vi "FRC-Traj-Lib-timer-test.vi"() -> ()   [LabVIEW 2019]
uses:
  <vilib>/Rock Robotics/WPI/ThirdParty/JAS_Junk/TrajLib/Trajectory_Library.lvlib
panel:
  in  "Tab Control":enum32{"Control Panel", "Logic"}(tab)
  in  "Reset TImer":bool
  in  "Stop Timer":bool
  in  "Start Timer":bool
  out "Trend":cluster{"CurrentTImer":dbl, "CurrentTImer":dbl}(graph)
  out "Expired":bool
  out "Timer 2":dbl
  out "Timer 1":dbl
  # "Timer Test"
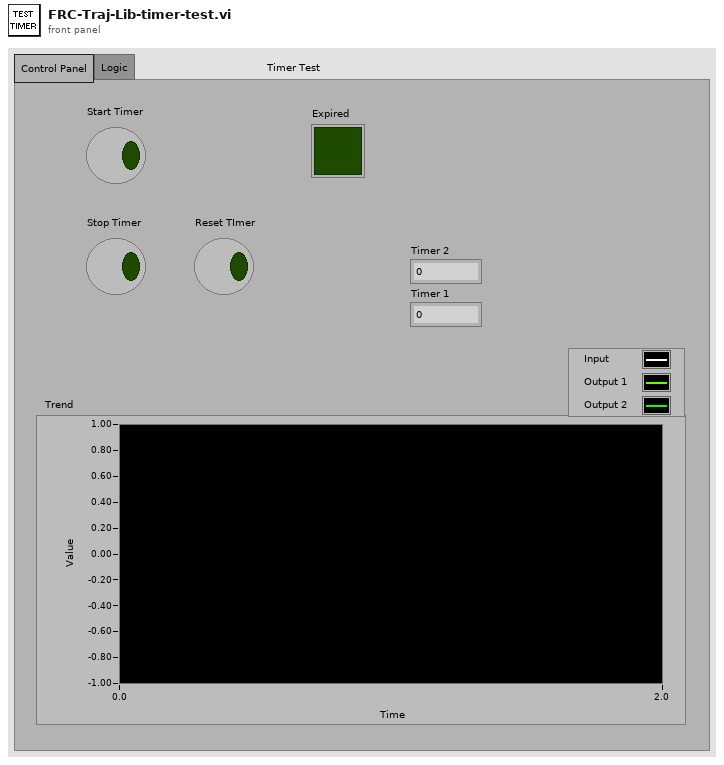
[diagram p1: front panel]
types:
  T1 = typedef "Trajectory_Library.lvlib/TIMER.ctl" = cluster{"StartTime":dbl, "Accumulated TIme":dbl, "Running":bool, "semaphore":T2}
  T2 = typedef "Semaphore RefNum" = refnum<k1>
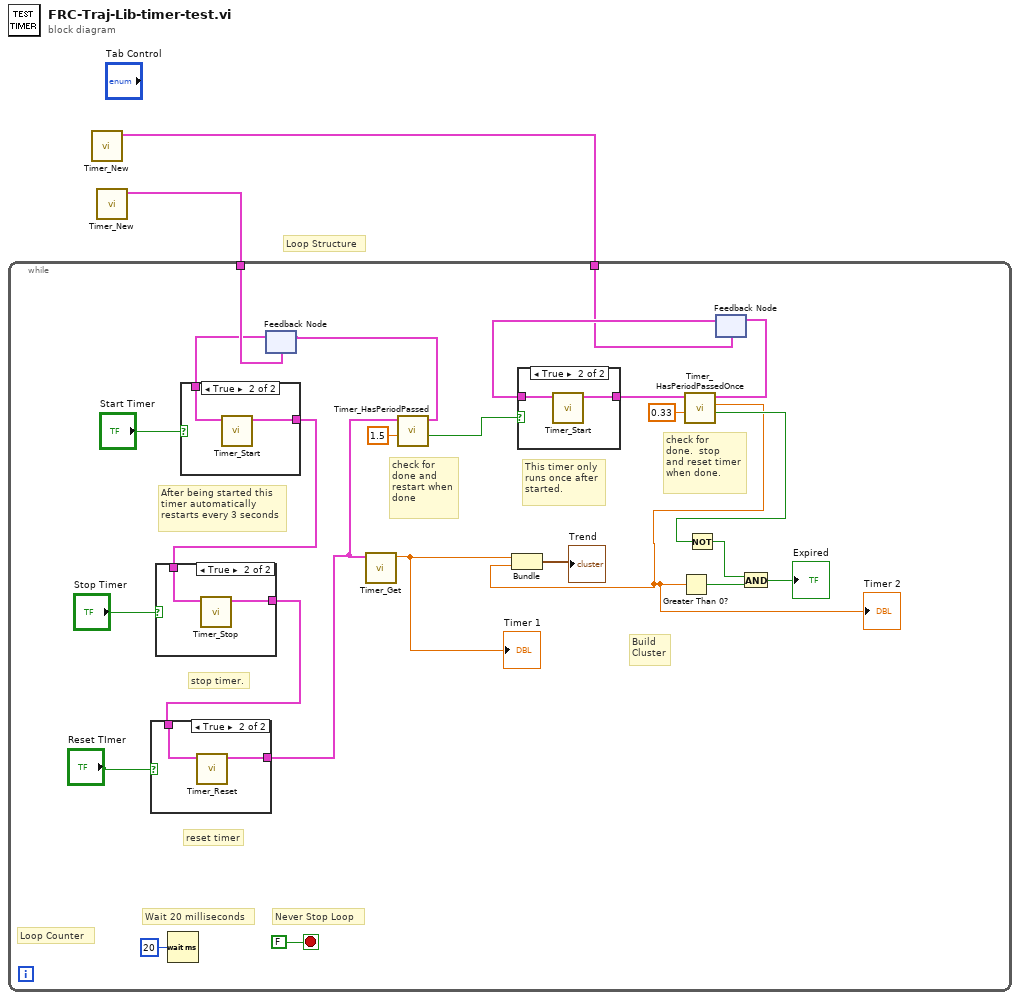
[diagram p0: block diagram]
diagram:
  # "Loop Structure"
  n1 = call <vilib>:"Timer_New.vi"() -> ("TIMER"=w1:T1)  [unwired: 11 in]
  n2 = call <vilib>:"Timer_New.vi"() -> ("TIMER"=w2:T1)  [unwired: 11 in]
  n3 = while {
    tunnel: w2 -> [w24]
    tunnel: w1 -> [w19]
    stop <- FALSE stop-if-true
    # "reset timer"
    # "stop timer."
    # "This timer only\nruns once after\nstarted."
    # "check for\ndone.  stop\nand reset timer\nwhen done."
    # "check for\ndone and\nrestart when\ndone"
    # "After being started this \ntimer automatically\nrestarts every 3 seconds"
    # "Build\nCluster"
    # "Loop Counter"
    # "Never Stop Loop"
    # "Wait 20 milliseconds"
    n4 = Wait (ms)(milliseconds to wait=u32 20) -> ()  [unwired: 1 out]
    n5 = feedback #1(w24) -> (w23:T1)
    n6 = case shown="True" "Start Timer" {
      tunnel: [w37 w39] -> w6
      tunnel: w23 -> [w37 w38]
      frame False {
      }
      frame True {
        n7 = call <vilib>:"Timer_Start.vi"("in Timer"=w38) -> ("out Timer"=w39:T1)  [unwired: 10 in]
      }
    }
    n8 = case shown="True" "Stop Timer" {
      tunnel: [w31 w33] -> w3
      tunnel: w6 -> [w31 w32]
      frame False {
      }
      frame True {
        n9 = call <vilib>:"Timer_Stop.vi"("in Timer"=w32) -> ("out Timer"=w33:T1)  [unwired: 10 in]
      }
    }
    n10 = case shown="True" "Reset TImer" {
      tunnel: [w28 w29] -> w4
      tunnel: w3 -> [w28 w30]
      frame False {
      }
      frame True {
        n11 = call <vilib>:"Timer_Reset.vi"("in TIMER"=w30) -> ("out TIMER"=w29:T1)  [unwired: 10 in]
      }
    }
    n12 = call <vilib>:"Timer_Get.vi"("TIMER"=w4) -> ("CurrentTImer"=w11:dbl)  [unwired: 10 in]
    "Timer 1" <- w11
    n13 = call <vilib>:"Timer_HasPeriodPassed.vi"("Period"=1.5, "in Timer"=w4) -> ("Expired"=w17:bool, "out Timer"=w22:T1)  [unwired: 7 in, 1 out]
    n14 = feedback-in #1(w22) -> ()
    n15 = feedback #2(w19) -> (w20:T1)
    n16 = case shown="True" w17 {
      tunnel: w20 -> [w34 w36]
      tunnel: [w34 w35] -> w12
      frame False {
      }
      frame True {
        n17 = call <vilib>:"Timer_Start.vi"("in Timer"=w36) -> ("out Timer"=w35:T1)  [unwired: 10 in]
      }
    }
    n18 = call <vilib>:"Timer_HasPeriodPassedOnce.vi"("Period"=0.33, "in Timer"=w12) -> ("Expired"=w16:bool, "CurrentTImer"=w8:dbl, "out Timer"=w9:T1)  [unwired: 7 in]
    "Timer 2" <- w8
    n19 = Bundle("CurrentTImer"=w11, "CurrentTImer"=w8) -> (→"Trend":cluster{"CurrentTImer":dbl, "CurrentTImer":dbl})  [unwired: 1 in]
    n20 = Greater Than 0?(x=w8) -> (x > 0?=w13:bool)
    n21 = Not(x=w16) -> (.not. x?=w14:bool)
    n22 = feedback-in #2(w9) -> ()
    n23 = And(x=w14, y=w13) -> (x .and. y?=→"Expired":bool)
  }
